vi "LVIS_Send.vi"(8 "Error In":errorcluster, 11 "Data In":string) -> (0 "Error Out":errorcluster)   [LabVIEW 2015]
doc: "Formats the event data to be sent to the Data Commander or backup file."
uses:
  Globals/LVIS_DcGlobals.vi
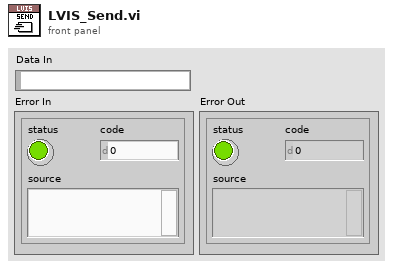
[diagram p1: front panel]
types:
  T1 = cluster{"ConnTimeout":string, "TxTimeout":string, "RxTimeout":string, "Port":string, "Map":string}
  T2 = typedef "LVIS_SAF Status.ctl" = u16
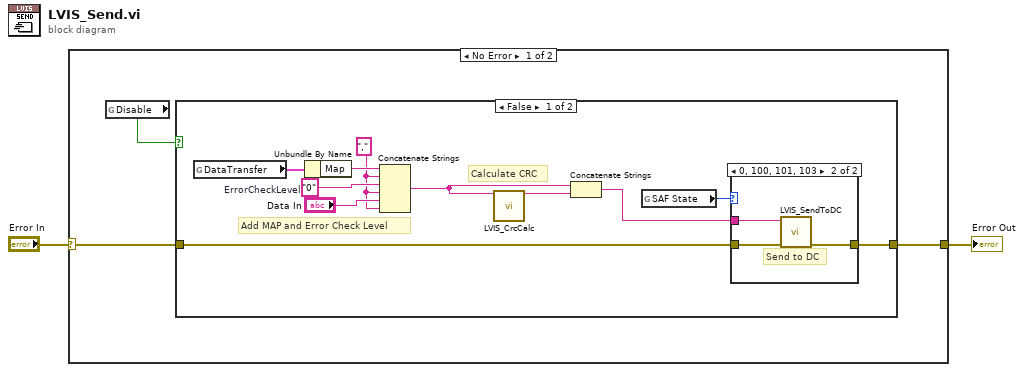
[diagram p0: block diagram]
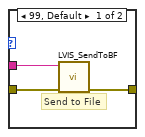
[diagram p2: hidden frame]
diagram:
  n1 = case shown="No Error" "Error In" {
    selector: "Error In" -> [w5 w24]
    tunnel: [w4 w24] -> w1
    frame No Error {
      n2 = global read "LVIS_DcGlobals.vi" "Disable"() -> (w3:bool)
      n3 = case shown="False" w3 {
        tunnel: w5 -> [w15 w23]
        tunnel: [w14 w23] -> w4
        frame False {
          w6 = ","
          w10 = "0"  # ErrorCheckLevel
          # "Add MAP and Error Check Level"
          # "Calculate CRC"
          n4 = global read "LVIS_DcGlobals.vi" "DataTransfer"() -> (w11:T1)
          n5 = Unbundle By Name(w11) -> ("Map"=w12:string)
          n6 = Concatenate Strings(w12, w6, w10, w6, "Data In", w6) -> (w7:string)
          n7 = call "LVIS_CrcCalc.vi"("String IN"=w7) -> ("CRC"=w13:string)  [unwired: 14 in]
          n8 = Concatenate Strings(w7, w13) -> (w9:string)
          n9 = global read "LVIS_DcGlobals.vi" "SAF State"() -> (w16:T2)
          n10 = case shown="0, 100, 101, 103" w16 {
            tunnel: w15 -> [w19 w22]
            tunnel: [w18 w21] -> w14
            tunnel: w9 -> [w17 w20]
            frame 99, Default {
              # "Send to File"
              n11 = call "LVIS_SendToBF.vi"("Error In"=w19, "Data"=w17) -> ("Error out"=w18:errorcluster)  [unwired: 9 in]
            }
            frame 0, 100, 101, 103 {
              # "Send to DC"
              n12 = call "LVIS_SendToDC.vi"("Error In"=w22, "Data"=w20) -> ("Error out"=w21:errorcluster)  [unwired: 7 in, 2 out]
            }
          }
        }
        frame True {
          # "The Data Commander has been disabled"
        }
      }
    }
    frame Error {
    }
  }
  "Error Out" <- w1
